vi "motortestMeng2.vi"() -> ()   [LabVIEW 2014]
panel:
  in  "MG17Motor":refnum<k7>(container)
  in  "stop":bool
  in  "Controller ID":i32=83829798
  out "Numeric":i32
  out "pfPosition":sgl
  out "GetPosition":i32
  in  "MG17Motor":refnum<k7>(container)
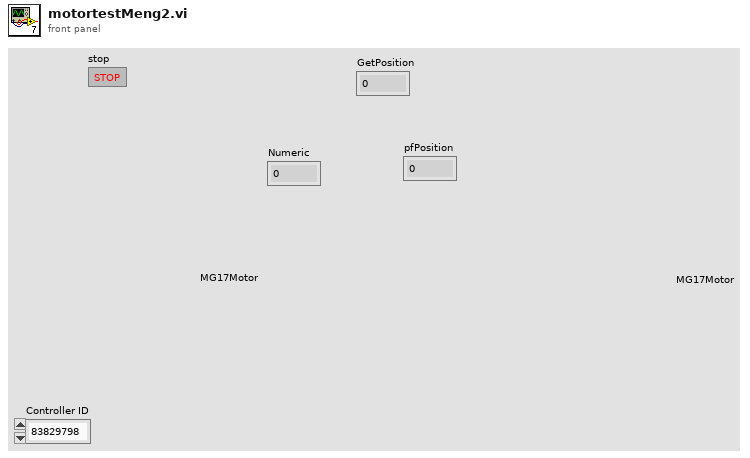
[diagram p1: front panel]
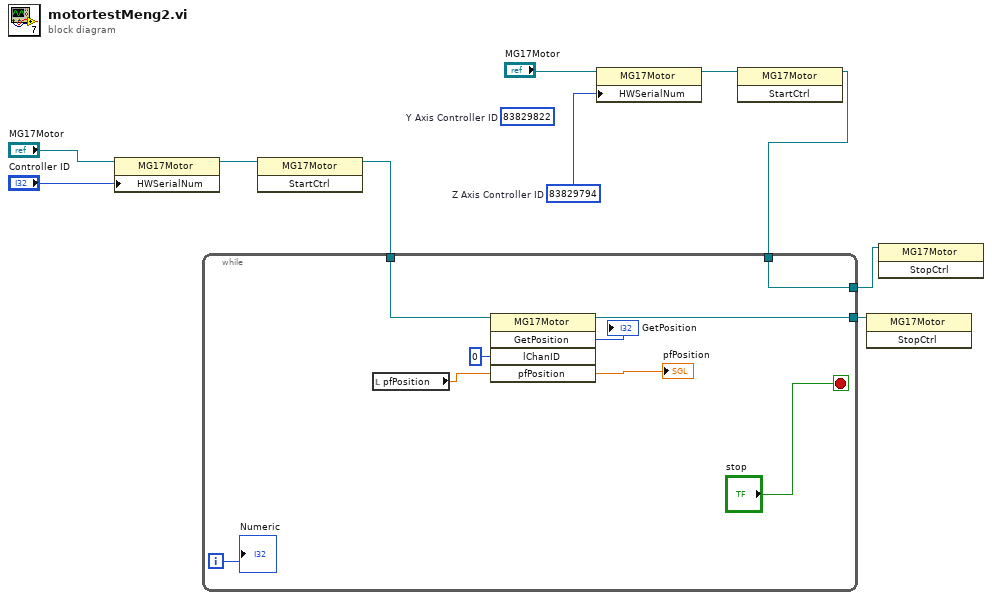
[diagram p0: block diagram]
diagram:
  w1 = 83829794  # Z Axis Controller ID
  (unwired) 83829822  # Y Axis Controller ID
  n1 = property class="MG17Motor"(reference="MG17Motor", "HWSerialNum"="Controller ID") -> (reference out=w7:refnum<k7>)  [unwired: 1 in, 1 out]
  n2 = invoke class="MG17Motor" method="StartCtrl"(reference=w7) -> (reference out=w6:refnum<k7>)  [unwired: 2 in, 2 out]
  n3 = property class="MG17Motor"(reference="MG17Motor", "HWSerialNum"=w1) -> (reference out=w2:refnum<k7>)  [unwired: 1 in, 1 out]
  n4 = invoke class="MG17Motor" method="StartCtrl"(reference=w2) -> (reference out=w4:refnum<k7>)  [unwired: 2 in, 2 out]
  n5 = while {
    tunnel: [w18] -> w10
    tunnel: w6 -> [w17]
    tunnel: [w12] -> w5
    tunnel: w4 -> [w12]
    i -> [w19]
    stop <- "stop" stop-if-true
    n6 = local read "pfPosition"() -> (w11:sgl)
    n7 = invoke class="MG17Motor" method="GetPosition"(reference=w17, "lChanID"=0, "pfPosition"=w11) -> (reference out=w18:refnum<k7>, "GetPosition"=→"GetPosition":i32, "pfPosition"=→"pfPosition":sgl)  [unwired: 2 in, 2 out]
    "Numeric" <- w19
  }
  n8 = invoke class="MG17Motor" method="StopCtrl"(reference=w10) -> ()  [unwired: 2 in, 3 out]
  n9 = invoke class="MG17Motor" method="StopCtrl"(reference=w5) -> ()  [unwired: 2 in, 3 out]
